vi "Medidor2.0.vi"() -> ()   [LabVIEW 2020]
uses:
  <vilib>/numeric/Random Number (Range) DBL.vi
panel:
  out "pot C":dbl[](array[numeric])
  out "V C":dbl[](array[numeric])
  out "IVVC C":dbl[](array[numeric])
  out "Potencia ativa C":dbl[](graph)
  out "Table 4":string[][](table)
  out "pot B":dbl[](array[numeric])
  out "V B":dbl[](array[numeric])
  out "I B":dbl[](array[numeric])
  out "Potencia ativa B":dbl[](graph)
  out "Table 3":string[][](table)
  out "pot A":dbl[](array[numeric])
  out "V A":dbl[](array[numeric])
  out "I A":dbl[](array[numeric])
  out "Potencia ativa A":dbl[](graph)
  out "fator de potencia":dbl
  in  "lower bound (0)":dbl
  in  "upper bound (100)":dbl=100.0
  out "Table 2":string[][](table)
  out "Table":string[][](table)
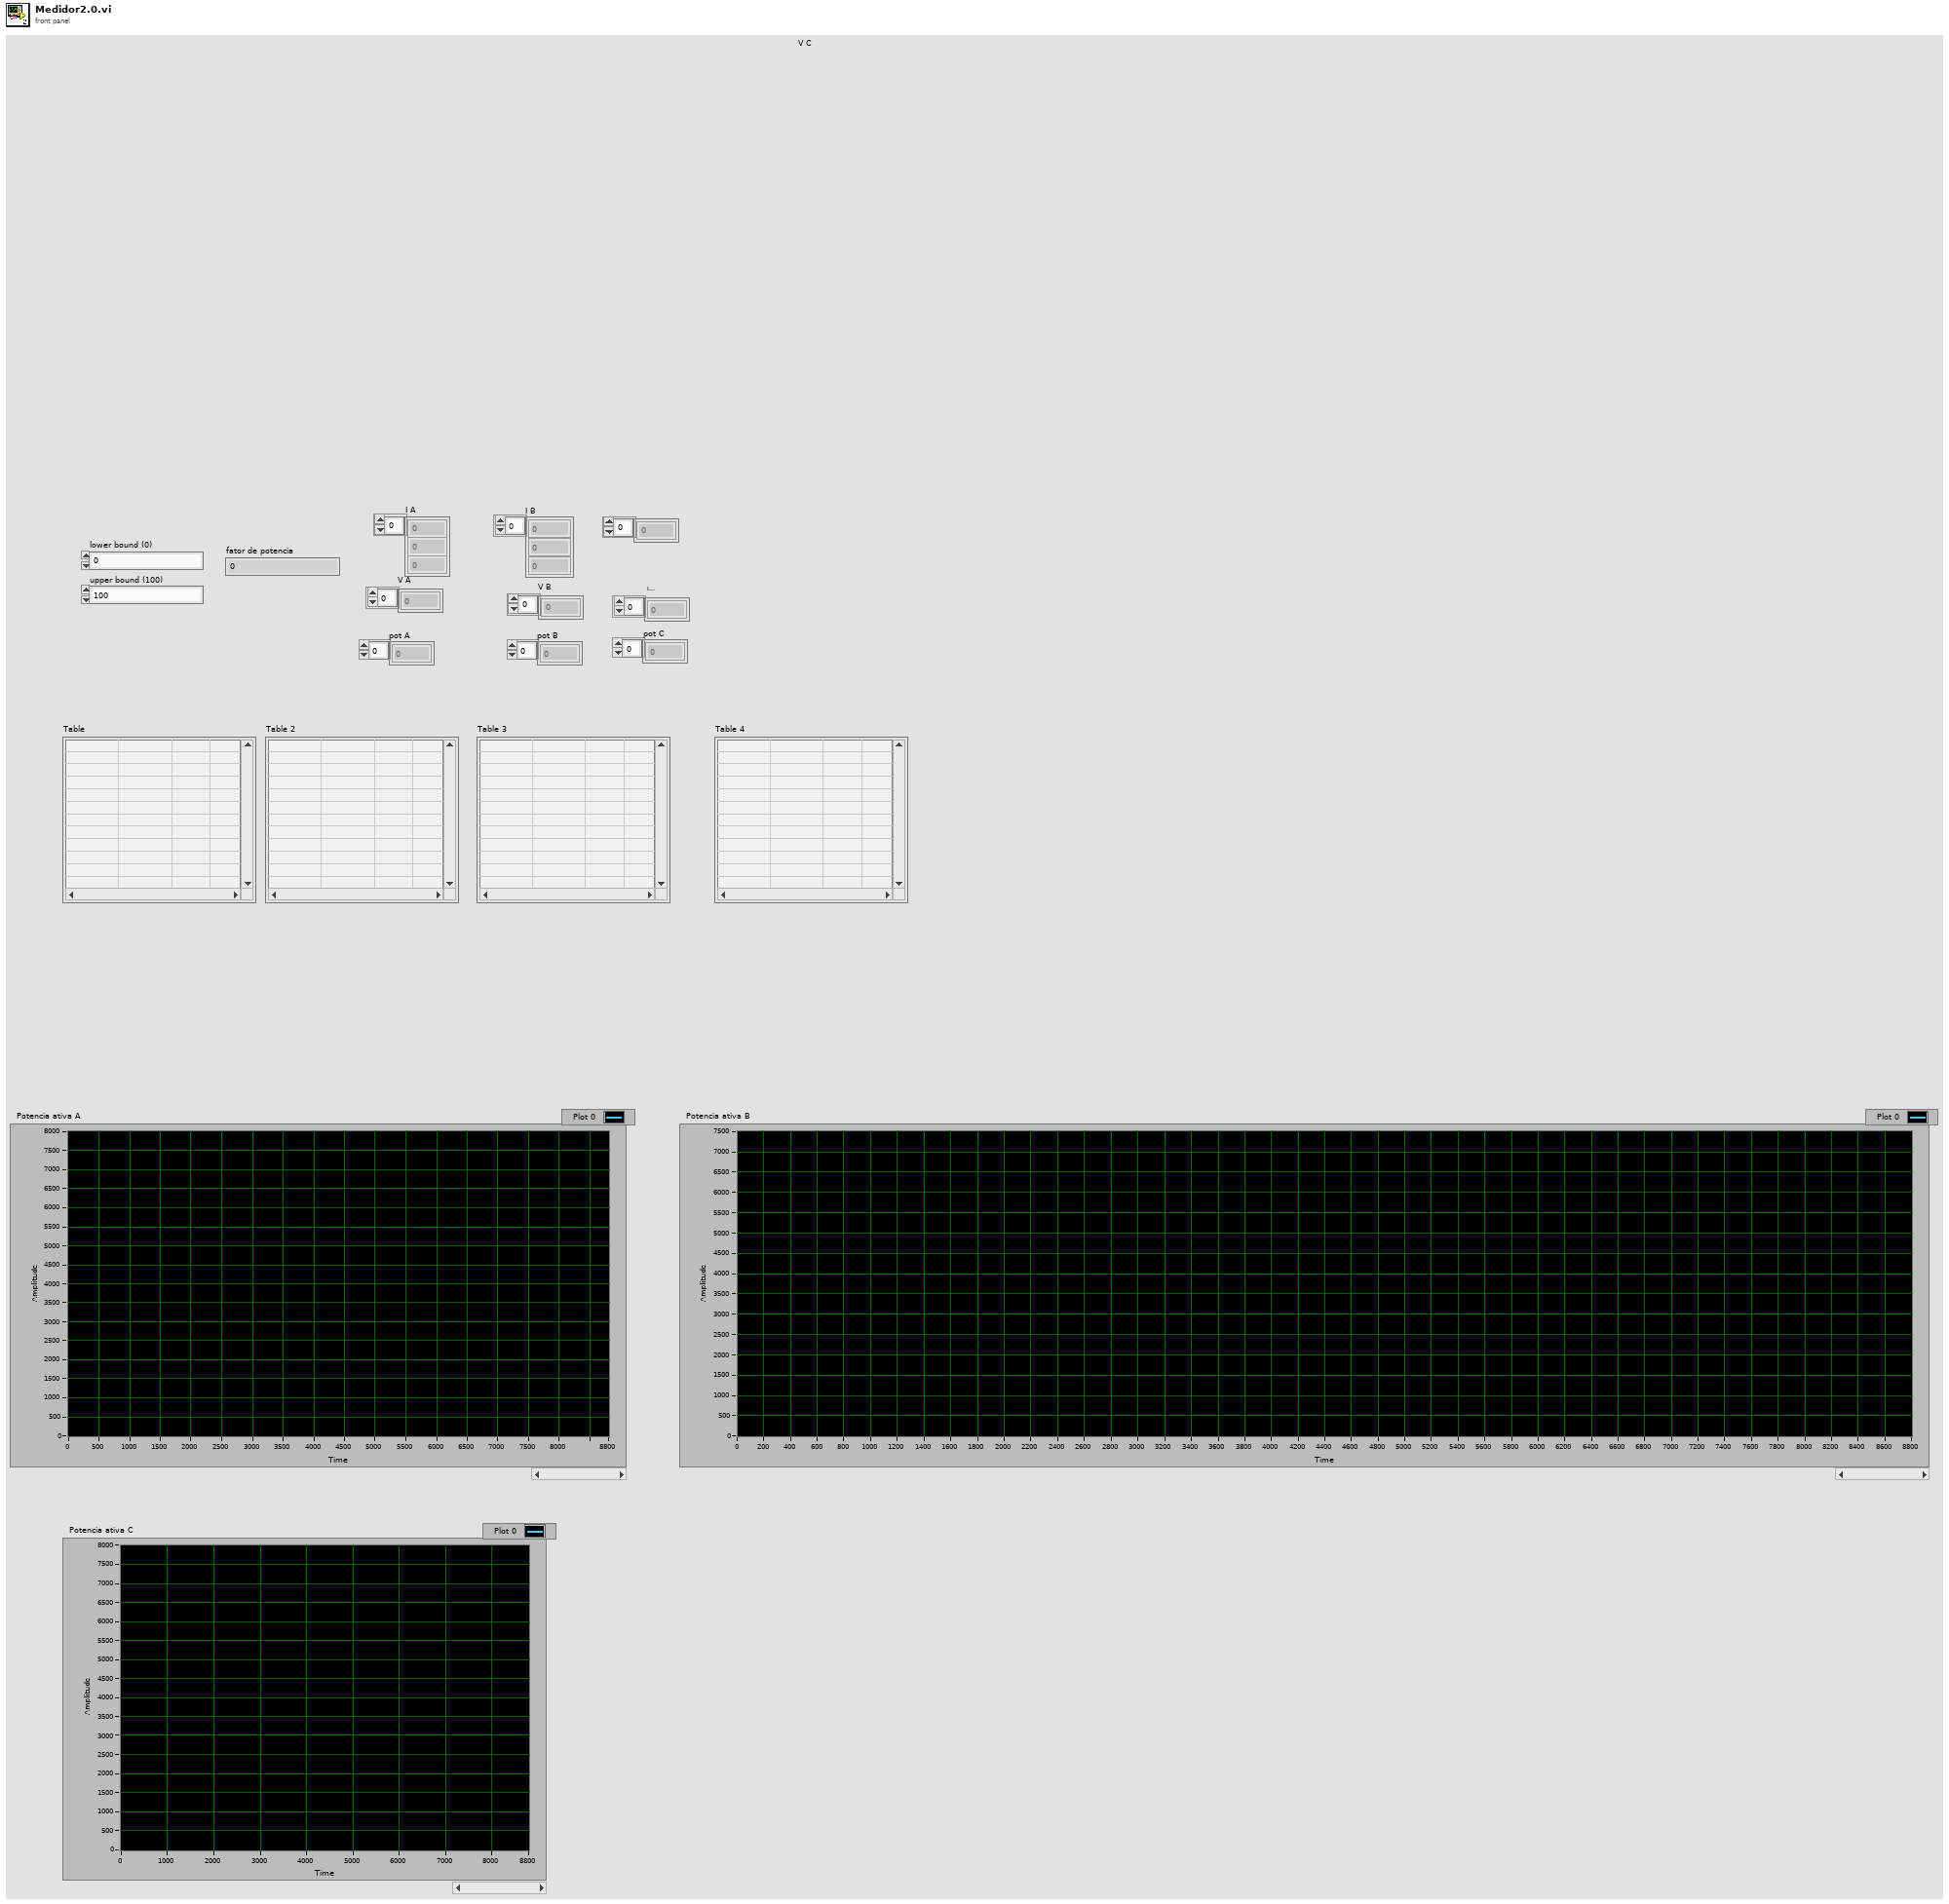
[diagram p1: front panel]
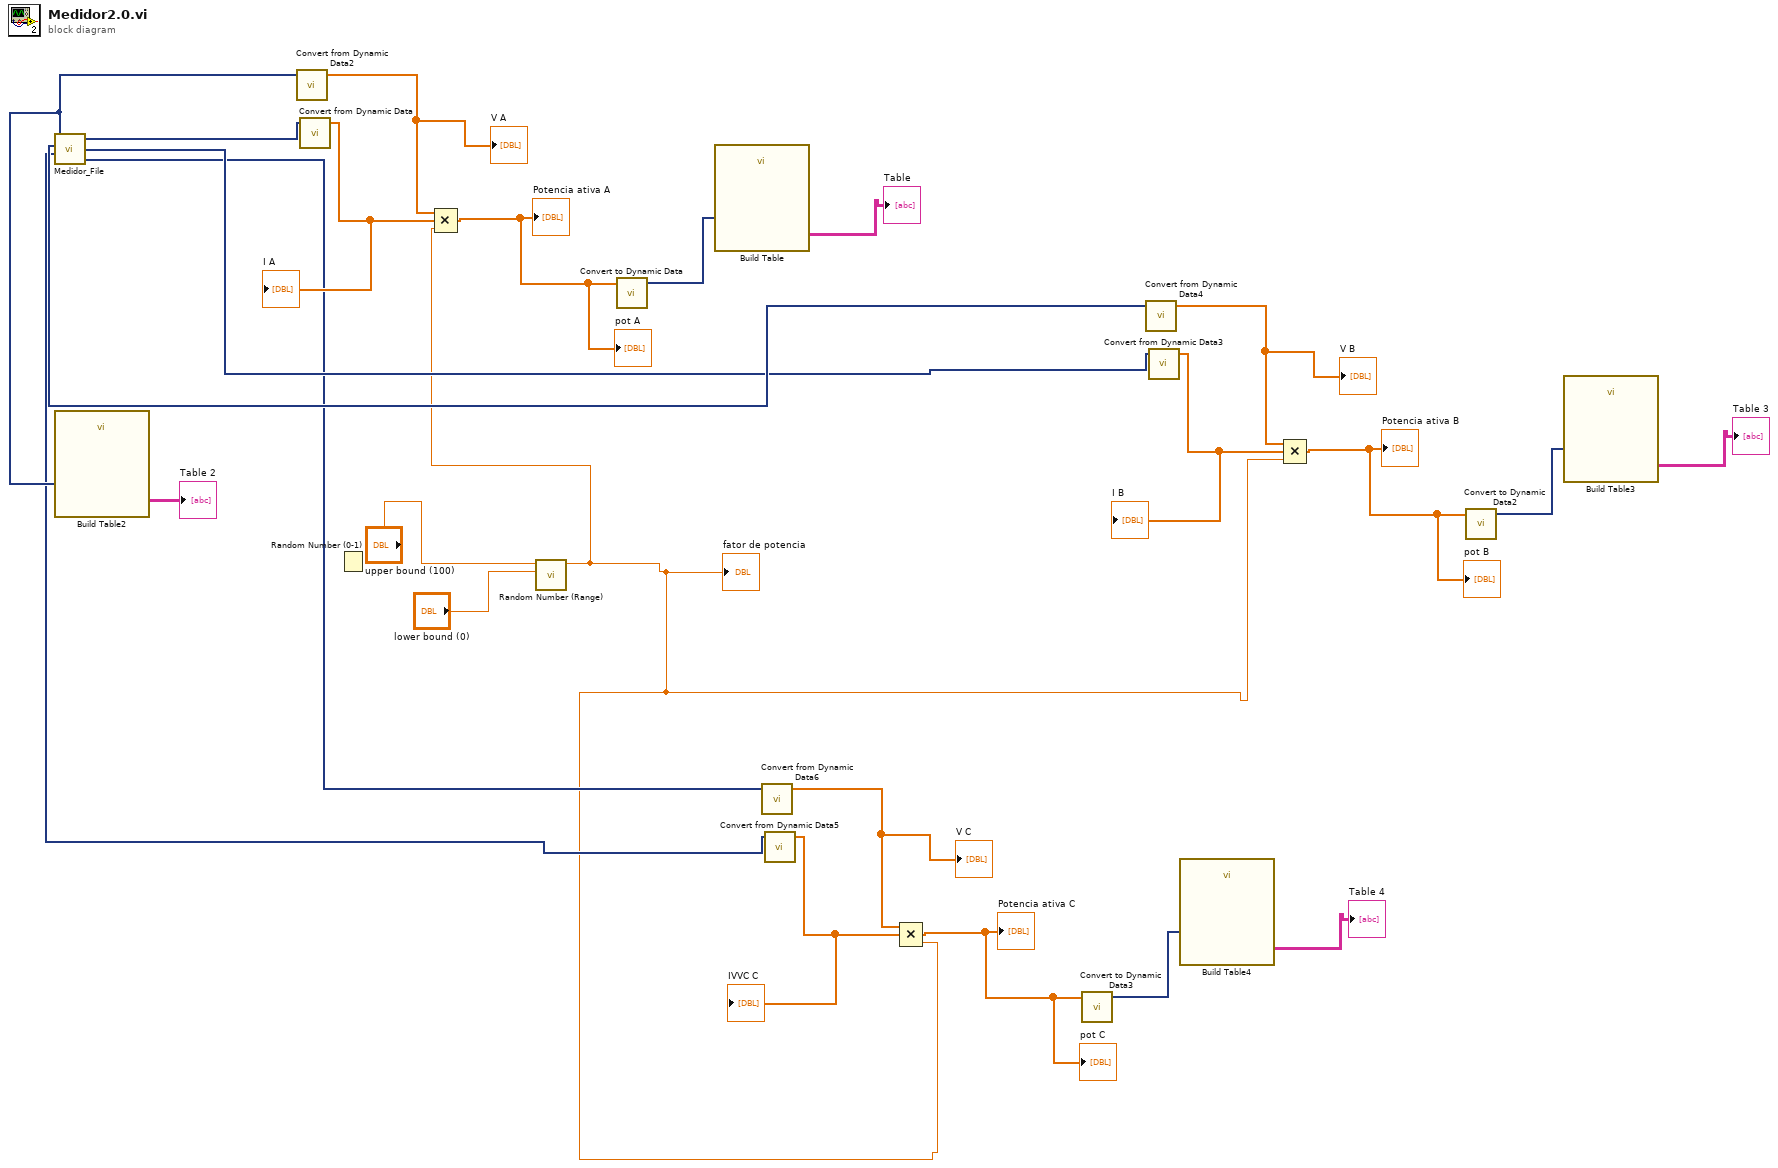
[diagram p0: block diagram]
diagram:
  n1 = call "Medidor_File.vi"() -> ("Corrente Fase C"=w3:dynamicdata, "Corrente Fase B"=w4:dynamicdata, "Corrente Fase A"=w22:dynamicdata, "Tensão Fase C"=w2:dynamicdata, "Tensão Fase B"=w5:dynamicdata, "Tensão Fase A"=w23:dynamicdata)  [unwired: 1 out]
  n2 = call "Build Table2"("Signals"=w23) -> ("Table"=→"Table 2":string[][])  [unwired: 4 in, 6 out]
  n3 = call "Convert from Dynamic Data2"("Dynamic Data Type"=w23) -> ("Array"=w18:dbl[])  [unwired: 3 in]
  "V A" <- w18
  n4 = call "Convert from Dynamic Data"("Dynamic Data Type"=w22) -> ("Array"=w19:dbl[])  [unwired: 3 in]
  "I A" <- w19
  n5 = Random Number (0-1)() -> ()  [unwired: 1 out]
  n6 = call-poly <vilib>:"Random Number (Range).vi"("lower bound (0)"="lower bound (0)", "upper bound (100)"="upper bound (100)") -> ("number"=w1:dbl)  [unwired: 9 in]
  "fator de potencia" <- w1
  n7 = Compound Arithmetic op=MULTIPLY(w18, w19, w1) -> (w16:dbl[])
  "Potencia ativa A" <- w16
  "pot A" <- w16
  n8 = call "Convert to Dynamic Data"("Array"=w16) -> ("Dynamic Data Type"=w20:dynamicdata)  [unwired: 3 in]
  n9 = call "Build Table"("Signals"=w20) -> ("Table"=→"Table":string[][])  [unwired: 4 in, 6 out]
  n10 = call "Convert from Dynamic Data6"("Dynamic Data Type"=w3) -> ("Array"=w8:dbl[])  [unwired: 3 in]
  "V C" <- w8
  n11 = call "Convert from Dynamic Data5"("Dynamic Data Type"=w2) -> ("Array"=w9:dbl[])  [unwired: 3 in]
  "IVVC C" <- w9
  n12 = Compound Arithmetic op=MULTIPLY(w8, w9, w1) -> (w6:dbl[])
  "Potencia ativa C" <- w6
  "pot C" <- w6
  n13 = call "Convert to Dynamic Data3"("Array"=w6) -> ("Dynamic Data Type"=w10:dynamicdata)  [unwired: 3 in]
  n14 = call "Convert from Dynamic Data4"("Dynamic Data Type"=w5) -> ("Array"=w13:dbl[])  [unwired: 3 in]
  "V B" <- w13
  n15 = call "Convert from Dynamic Data3"("Dynamic Data Type"=w4) -> ("Array"=w14:dbl[])  [unwired: 3 in]
  "I B" <- w14
  n16 = call "Build Table4"("Signals"=w10) -> ("Table"=→"Table 4":string[][])  [unwired: 4 in, 6 out]
  n17 = Compound Arithmetic op=MULTIPLY(w13, w14, w1) -> (w11:dbl[])
  "Potencia ativa B" <- w11
  "pot B" <- w11
  n18 = call "Convert to Dynamic Data2"("Array"=w11) -> ("Dynamic Data Type"=w15:dynamicdata)  [unwired: 3 in]
  n19 = call "Build Table3"("Signals"=w15) -> ("Table"=→"Table 3":string[][])  [unwired: 4 in, 6 out]
